vi "JL_Parse_Snapshot.vi"(0 "GEA2 Reference In":refnum<k24>, 5 "GEA Inputs":T2={"Source"=228, "Destination"=192} {"Destination" format="%.0x"; "Source" format="%.0x"}, 7 "SnapShot Location":T1={"ERD Number"=57629, "Data Type"=enum."string"} {"ERD Number" format="%.0x"}, 11 "Error In":errorcluster, 12 "Low Level Tries":u8=5) -> (4 "GEA2 Reference Out":refnum<k24>, 8 "Fault Snapshot":string[](array[string]), 15 "Error Out":errorcluster)   [LabVIEW 2023]
uses:
  D:/Common/LabVIEW GEA2 Toolkit/source/GEA3 DLL Source/GeaCommunication.dll
  Common/LabVIEW GEA2 Toolkit/source/GEA3 DLL Source/GeaCommunication.dll
  Common/LabVIEW GEA2 Toolkit/GEA3/type defs/Source_Destination.ctl
  Common/LabVIEW GEA2 Toolkit/GEA3/type defs/ERD Read Data In.ctl
  Common/LabVIEW GEA2 Toolkit/GEA3/library/GEA2_Toolkit.lvlib
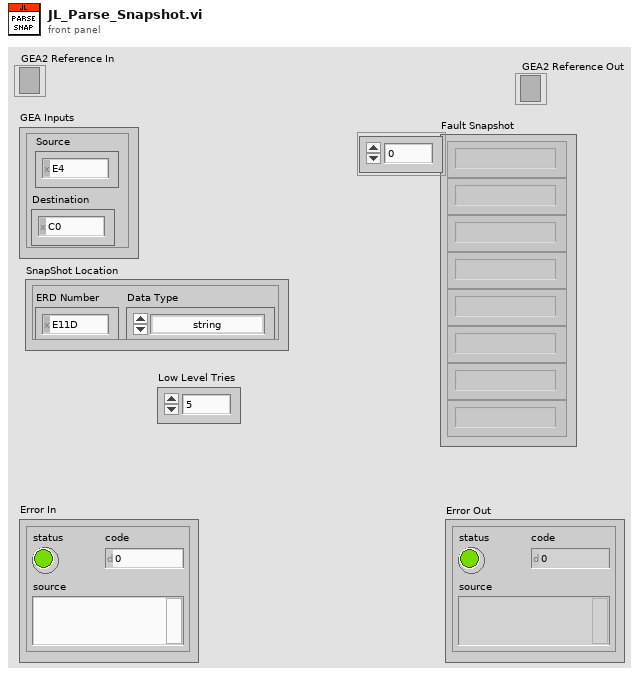
[diagram p1: front panel]
types:
  T1 = typedef "ERD Read Data In.ctl" = cluster{"ERD Number":u16, "Data Type":enum16{"string", "boolean", "uint8_t", "uint16_t", "uint32_t", "uint64_t", "int8_t", "int16_t", "int32_t", "int64_t"}}
  T2 = typedef "Source_Destination.ctl" = cluster{"Source":u8, "Destination":u8}
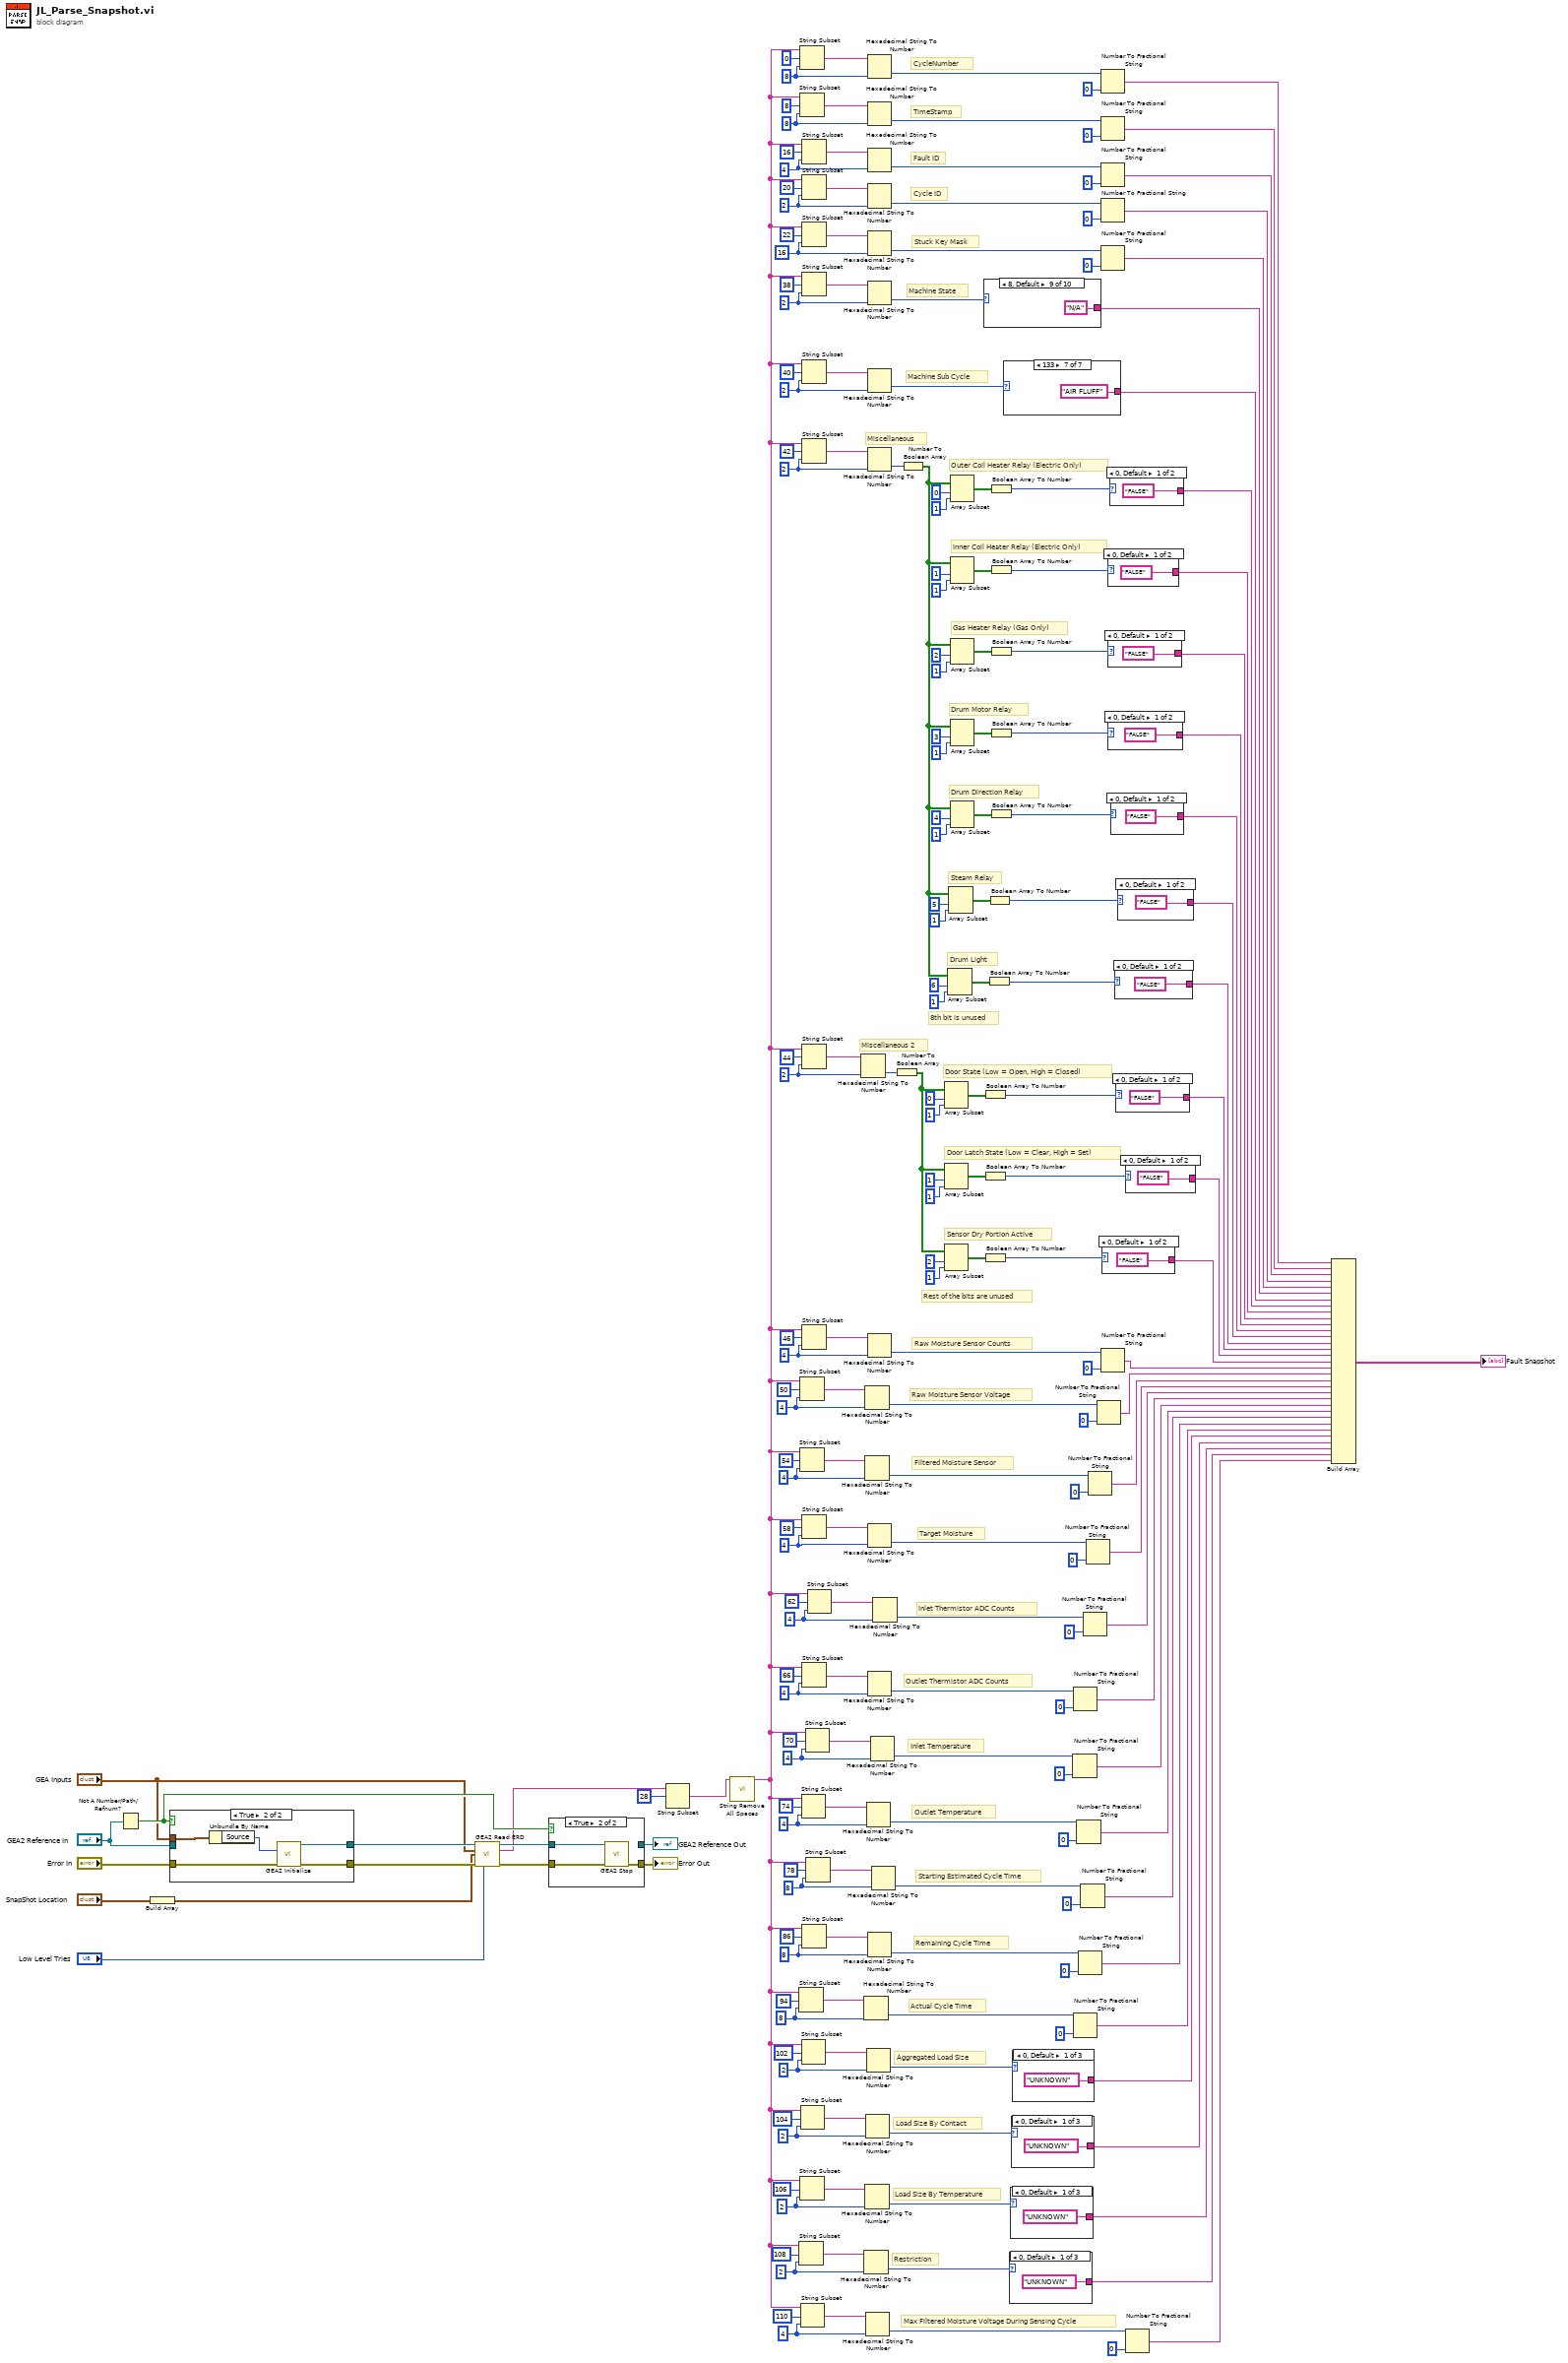
[diagram p0: block diagram]
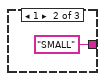
[diagram p2: hidden frame]
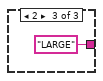
[diagram p3: hidden frame]
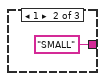
[diagram p4: hidden frame]
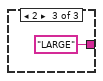
[diagram p5: hidden frame]
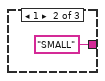
[diagram p6: hidden frame]
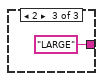
[diagram p7: hidden frame]
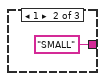
[diagram p8: hidden frame]
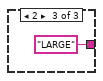
[diagram p9: hidden frame]
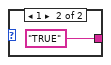
[diagram p10: hidden frame]
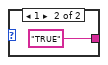
[diagram p11: hidden frame]
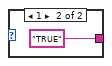
[diagram p12: hidden frame]
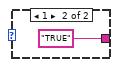
[diagram p13: hidden frame]
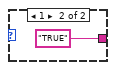
[diagram p14: hidden frame]
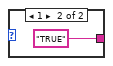
[diagram p15: hidden frame]
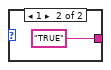
[diagram p16: hidden frame]
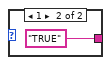
[diagram p17: hidden frame]
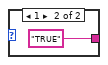
[diagram p18: hidden frame]
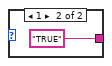
[diagram p19: hidden frame]
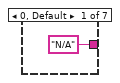
[diagram p20: hidden frame]
diagram:
  w14 = 4 ("length (rest)")
  w18 = 2 ("length (rest)")
  w22 = 2 ("length (rest)")
  w26 = 2 ("length (rest)")
  w31 = 2 ("length (rest)")
  w122 = 8 ("length (rest)")
  w123 = 4 ("length (rest)")
  w130 = 4 ("length (rest)")
  w146 = 8 ("length (rest)")
  w147 = 8 ("length (rest)")
  w148 = 4 ("length (rest)")
  w149 = 4 ("length (rest)")
  w150 = 4 ("length (rest)")
  w151 = 4 ("length (rest)")
  w152 = 4 ("length (rest)")
  w153 = 4 ("length (rest)")
  w63 = 2 ("length (rest)")
  w154 = 2 ("length (rest)")
  w155 = 2 ("length (rest)")
  w156 = 2 ("length (rest)")
  w157 = 16 ("length (rest)")
  w158 = 2 ("length (rest)")
  w159 = 4 ("length (rest)")
  w160 = 8 ("length (rest)")
  w161 = 8 ("length (rest)")
  # "Max Filtered Moisture Voltage During Sensing Cycle"
  # "Restriction"
  # "Load Size By Temperature"
  # "Load Size By Contact"
  # "Aggregated Load Size"
  # "Actual Cycle Time"
  # "Remaining Cycle Time"
  # "Starting Estimated Cycle Time"
  # "Outlet Temperature"
  # "Inlet Temperature"
  # "Outlet Thermistor ADC Counts"
  # "Inlet Thermistor ADC Counts"
  # "Target Moisture"
  # "Filtered Moisture Sensor"
  # "Rest of the bits are unused"
  # "Sensor Dry Portion Active"
  # "Door Latch State (Low = Clear, High = Set)"
  # "Door State (Low = Open, High = Closed)"
  # "Miscellaneous 2"
  # "8th bit is unused"
  # "Drum Light"
  # "Steam Relay"
  # "Drum Direction Relay"
  # "Drum Motor Relay"
  # "Gas Heater Relay (Gas Only)"
  # "Inner Coil Heater Relay (Electric Only)"
  # "Outer Coil Heater Relay (Electric Only)"
  # "Stuck Key Mask"
  # "Raw Moisture Sensor Counts"
  # "Raw Moisture Sensor Voltage"
  # "Miscellaneous"
  # "Machine Sub Cycle"
  # "Cycle ID"
  # "Fault ID"
  # "Machine State"
  # "TimeStamp"
  # "CycleNumber"
  n1 = Not A Number/Path/Refnum?(number/path/refnum="GEA2 Reference In") -> (NaN/Path/Refnum?=w142:bool)
  n2 = Build Array("SnapShot Location") -> (w1:T1[])
  n3 = case shown="True" w142 {
    tunnel: "GEA Inputs" -> [_ w217]
    tunnel: "Error In" -> [w212 w216]
    tunnel: [w212 w215] -> w136
    tunnel: [w211 w214] -> w140
    tunnel: "GEA2 Reference In" -> [w211 _]
    frame False {
    }
    frame True {
      n4 = Unbundle By Name(w217) -> ("Source"=w213:u8)
      n5 = call "GEA2 Initialize.vi"("Source Address"=w213, "error in"=w216) -> ("GEA2 Reference Out"=w214:refnum<k24>, "error out"=w215:errorcluster)  [unwired: 10 in, 2 out]
    }
  }
  n6 = call "GEA2 Read ERD.vi"("GEA2 Reference In"=w140, "GEA Inputs"="GEA Inputs", "Read ERD List"=w1, "Error In"=w136, "Low Level Tries"="Low Level Tries") -> ("GEA2 Reference Out"=w138:refnum<k24>, "Raw Data Out"=w131:string, "Error Out"=w137:errorcluster)  [unwired: 7 in, 1 out]
  n7 = case shown="True" w142 {
    tunnel: [w218 w222] -> w143
    tunnel: [w219 _] -> w141
    tunnel: w138 -> [w219 w220]
    tunnel: w137 -> [w218 w221]
    frame False {
    }
    frame True {
      n8 = call "GEA2 Stop.vi"("GEA2 Reference In"=w220, "Error In"=w221) -> ("Error Out"=w222:errorcluster)  [unwired: 13 in]
    }
  }
  "Error Out" <- w143
  "GEA2 Reference Out" <- w141
  n9 = String Subset(string=w131, offset (0)=28) -> (substring=w132:string)  [unwired: 1 in]
  n10 = call "String Remove All Spaces.vi"("Input String"=w132) -> ("Spaces Removed"=w9:string)  [unwired: 13 in, 1 out]
  n11 = String Subset(string=w9, offset (0)=94, length (rest)=w122) -> (substring=w121:string)
  n12 = String Subset(string=w9, offset (0)=108, length (rest)=w18) -> (substring=w17:string)
  n13 = String Subset(string=w9, offset (0)=0, length (rest)=w161) -> (substring=w210:string)
  n14 = String Subset(string=w9, offset (0)=8, length (rest)=w160) -> (substring=w209:string)
  n15 = String Subset(string=w9, offset (0)=50, length (rest)=w130) -> (substring=w129:string)
  n16 = String Subset(string=w9, offset (0)=54, length (rest)=w123) -> (substring=w124:string)
  n17 = String Subset(string=w9, offset (0)=106, length (rest)=w22) -> (substring=w21:string)
  n18 = String Subset(string=w9, offset (0)=104, length (rest)=w26) -> (substring=w25:string)
  n19 = String Subset(string=w9, offset (0)=110, length (rest)=w14) -> (substring=w13:string)
  n20 = String Subset(string=w9, offset (0)=74, length (rest)=w148) -> (substring=w184:string)
  n21 = String Subset(string=w9, offset (0)=102, length (rest)=w31) -> (substring=w30:string)
  n22 = String Subset(string=w9, offset (0)=16, length (rest)=w159) -> (substring=w208:string)
  n23 = String Subset(string=w9, offset (0)=20, length (rest)=w158) -> (substring=w207:string)
  n24 = String Subset(string=w9, offset (0)=22, length (rest)=w157) -> (substring=w196:string)
  n25 = String Subset(string=w9, offset (0)=38, length (rest)=w156) -> (substring=w197:string)
  n26 = String Subset(string=w9, offset (0)=40, length (rest)=w155) -> (substring=w198:string)
  n27 = String Subset(string=w9, offset (0)=42, length (rest)=w154) -> (substring=w3:string)
  n28 = String Subset(string=w9, offset (0)=44, length (rest)=w63) -> (substring=w64:string)
  n29 = String Subset(string=w9, offset (0)=46, length (rest)=w153) -> (substring=w185:string)
  n30 = String Subset(string=w9, offset (0)=58, length (rest)=w152) -> (substring=w195:string)
  n31 = String Subset(string=w9, offset (0)=66, length (rest)=w150) -> (substring=w193:string)
  n32 = String Subset(string=w9, offset (0)=86, length (rest)=w146) -> (substring=w182:string)
  n33 = String Subset(string=w9, offset (0)=70, length (rest)=w149) -> (substring=w192:string)
  n34 = String Subset(string=w9, offset (0)=78, length (rest)=w147) -> (substring=w183:string)
  n35 = String Subset(string=w9, offset (0)=62, length (rest)=w151) -> (substring=w194:string)
  n36 = Hexadecimal String To Number(string=w64, default (0uL)=w63) -> (number=w78:i32)  [unwired: 1 in, 1 out]
  n37 = Hexadecimal String To Number(string=w121, default (0uL)=w122) -> (number=w32:i32)  [unwired: 1 in, 1 out]
  n38 = Hexadecimal String To Number(string=w17, default (0uL)=w18) -> (number=w15:i32)  [unwired: 1 in, 1 out]
  n39 = Hexadecimal String To Number(string=w129, default (0uL)=w130) -> (number=w126:i32)  [unwired: 1 in, 1 out]
  n40 = Hexadecimal String To Number(string=w124, default (0uL)=w123) -> (number=w56:i32)  [unwired: 1 in, 1 out]
  n41 = Hexadecimal String To Number(string=w21, default (0uL)=w22) -> (number=w19:i32)  [unwired: 1 in, 1 out]
  n42 = Hexadecimal String To Number(string=w25, default (0uL)=w26) -> (number=w23:i32)  [unwired: 1 in, 1 out]
  n43 = Hexadecimal String To Number(string=w13, default (0uL)=w14) -> (number=w10:i32)  [unwired: 1 in, 1 out]
  n44 = Hexadecimal String To Number(string=w184, default (0uL)=w148) -> (number=w41:i32)  [unwired: 1 in, 1 out]
  n45 = Hexadecimal String To Number(string=w30, default (0uL)=w31) -> (number=w27:i32)  [unwired: 1 in, 1 out]
  n46 = Hexadecimal String To Number(string=w210, default (0uL)=w161) -> (number=w173:i32)  [unwired: 1 in, 1 out]
  n47 = Hexadecimal String To Number(string=w209, default (0uL)=w160) -> (number=w174:i32)  [unwired: 1 in, 1 out]
  n48 = Hexadecimal String To Number(string=w208, default (0uL)=w159) -> (number=w162:i32)  [unwired: 1 in, 1 out]
  n49 = Hexadecimal String To Number(string=w207, default (0uL)=w158) -> (number=w171:i32)  [unwired: 1 in, 1 out]
  n50 = Hexadecimal String To Number(string=w196, default (0uL)=w157) -> (number=w172:i32)  [unwired: 1 in, 1 out]
  n51 = Hexadecimal String To Number(string=w197, default (0uL)=w156) -> (number=w119:i32)  [unwired: 1 in, 1 out]
  n52 = Hexadecimal String To Number(string=w198, default (0uL)=w155) -> (number=w117:i32)  [unwired: 1 in, 1 out]
  n53 = Hexadecimal String To Number(string=w3, default (0uL)=w154) -> (number=w115:i32)  [unwired: 1 in, 1 out]
  n54 = Hexadecimal String To Number(string=w185, default (0uL)=w153) -> (number=w170:i32)  [unwired: 1 in, 1 out]
  n55 = Hexadecimal String To Number(string=w195, default (0uL)=w152) -> (number=w53:i32)  [unwired: 1 in, 1 out]
  n56 = Hexadecimal String To Number(string=w193, default (0uL)=w150) -> (number=w47:i32)  [unwired: 1 in, 1 out]
  n57 = Hexadecimal String To Number(string=w182, default (0uL)=w146) -> (number=w35:i32)  [unwired: 1 in, 1 out]
  n58 = Hexadecimal String To Number(string=w192, default (0uL)=w149) -> (number=w44:i32)  [unwired: 1 in, 1 out]
  n59 = Hexadecimal String To Number(string=w183, default (0uL)=w147) -> (number=w38:i32)  [unwired: 1 in, 1 out]
  n60 = Hexadecimal String To Number(string=w194, default (0uL)=w151) -> (number=w50:i32)  [unwired: 1 in, 1 out]
  n61 = Number To Boolean Array(number=w78) -> (Boolean array=w65:bool[])
  n62 = Number To Boolean Array(number=w115) -> (Boolean array=w86:bool[])
  n63 = Array Subset(array=w65, index=0, length=1) -> (w68:bool[])
  n64 = Array Subset(array=w65, index=1, length=1) -> (w67:bool[])
  n65 = Array Subset(array=w65, index=2, length=1) -> (w66:bool[])
  n66 = Array Subset(array=w86, index=6, length=1) -> (w87:bool[])
  n67 = Array Subset(array=w86, index=5, length=1) -> (w91:bool[])
  n68 = Array Subset(array=w86, index=0, length=1) -> (w99:bool[])
  n69 = Array Subset(array=w86, index=1, length=1) -> (w98:bool[])
  n70 = Array Subset(array=w86, index=2, length=1) -> (w97:bool[])
  n71 = Array Subset(array=w86, index=3, length=1) -> (w96:bool[])
  n72 = Array Subset(array=w86, index=4, length=1) -> (w95:bool[])
  n73 = case shown="8, Default" w119 {
    tunnel: ["IDLE" "STANDBY" "RUN" "PAUSE" "EOC" "DSM DELAY RUN" "DELAY RUN" "DELAY PAUSE" "N/A" "CLEAN SPEAK"] -> w118
    frame 0 {
    }
    frame 1 {
    }
    frame 2 {
    }
    frame 3 {
    }
    frame 4 {
    }
    frame 5 {
    }
    frame 6 {
    }
    frame 7 {
    }
    frame 8, Default {
    }
    frame 128 {
    }
  }
  n74 = Boolean Array To Number(Boolean array=w68) -> (number=w77:u32)
  n75 = Boolean Array To Number(Boolean array=w67) -> (number=w76:u32)
  n76 = Boolean Array To Number(Boolean array=w66) -> (number=w75:u32)
  n77 = Boolean Array To Number(Boolean array=w87) -> (number=w90:u32)
  n78 = Boolean Array To Number(Boolean array=w91) -> (number=w94:u32)
  n79 = Boolean Array To Number(Boolean array=w99) -> (number=w114:u32)
  n80 = Boolean Array To Number(Boolean array=w98) -> (number=w113:u32)
  n81 = Boolean Array To Number(Boolean array=w97) -> (number=w112:u32)
  n82 = Boolean Array To Number(Boolean array=w96) -> (number=w111:u32)
  n83 = Boolean Array To Number(Boolean array=w95) -> (number=w110:u32)
  n84 = case shown="133" w117 {
    tunnel: ["N/A" "DRYING" "MIST STEAM" "COOL DOWN" "EXTENDED TUMBLE" "DAMP" "AIR FLUFF"] -> w116
    frame 0, Default {
    }
    frame 128 {
    }
    frame 129 {
    }
    frame 130 {
    }
    frame 131 {
    }
    frame 132 {
    }
    frame 133 {
    }
  }
  n85 = case shown="0, Default" w15 {
    tunnel: ["UNKNOWN" "SMALL" "LARGE"] -> w5
    frame 0, Default {
    }
    frame 1 {
    }
    frame 2 {
    }
  }
  n86 = case shown="0, Default" w19 {
    tunnel: ["UNKNOWN" "SMALL" "LARGE"] -> w6
    frame 0, Default {
    }
    frame 1 {
    }
    frame 2 {
    }
  }
  n87 = case shown="0, Default" w23 {
    tunnel: ["UNKNOWN" "SMALL" "LARGE"] -> w7
    frame 0, Default {
    }
    frame 1 {
    }
    frame 2 {
    }
  }
  n88 = case shown="0, Default" w27 {
    tunnel: ["UNKNOWN" "SMALL" "LARGE"] -> w8
    frame 0, Default {
    }
    frame 1 {
    }
    frame 2 {
    }
  }
  n89 = Number To Fractional String(number=w44, precision (6)=i16 0) -> (F-format string=w43:string)  [unwired: 2 in]
  n90 = Number To Fractional String(number=w47, precision (6)=i16 0) -> (F-format string=w46:string)  [unwired: 2 in]
  n91 = Number To Fractional String(number=w32, precision (6)=i16 0) -> (F-format string=w28:string)  [unwired: 2 in]
  n92 = Number To Fractional String(number=w41, precision (6)=i16 0) -> (F-format string=w40:string)  [unwired: 2 in]
  n93 = Number To Fractional String(number=w35, precision (6)=i16 0) -> (F-format string=w34:string)  [unwired: 2 in]
  n94 = Number To Fractional String(number=w38, precision (6)=i16 0) -> (F-format string=w37:string)  [unwired: 2 in]
  n95 = Number To Fractional String(number=w50, precision (6)=i16 0) -> (F-format string=w49:string)  [unwired: 2 in]
  n96 = Number To Fractional String(number=w53, precision (6)=i16 0) -> (F-format string=w52:string)  [unwired: 2 in]
  n97 = Number To Fractional String(number=w56, precision (6)=i16 0) -> (F-format string=w55:string)  [unwired: 2 in]
  n98 = Number To Fractional String(number=w126, precision (6)=i16 0) -> (F-format string=w58:string)  [unwired: 2 in]
  n99 = Number To Fractional String(number=w173, precision (6)=u32 0) -> (F-format string=w169:string)  [unwired: 2 in]
  n100 = Number To Fractional String(number=w174, precision (6)=u32 0) -> (F-format string=w168:string)  [unwired: 2 in]
  n101 = Number To Fractional String(number=w162, precision (6)=u32 0) -> (F-format string=w163:string)  [unwired: 2 in]
  n102 = Number To Fractional String(number=w171, precision (6)=u32 0) -> (F-format string=w167:string)  [unwired: 2 in]
  n103 = Number To Fractional String(number=w172, precision (6)=i16 0) -> (F-format string=w166:string)  [unwired: 2 in]
  n104 = Number To Fractional String(number=w170, precision (6)=i16 0) -> (F-format string=w59:string)  [unwired: 2 in]
  n105 = case shown="0, Default" w75 {
    tunnel: ["FALSE" "TRUE"] -> w60
    frame 0, Default {
    }
    frame 1 {
    }
  }
  n106 = case shown="0, Default" w113 {
    tunnel: ["FALSE" "TRUE"] -> w84
    frame 0, Default {
    }
    frame 1 {
    }
  }
  n107 = case shown="0, Default" w112 {
    tunnel: ["FALSE" "TRUE"] -> w83
    frame 0, Default {
    }
    frame 1 {
    }
  }
  n108 = case shown="0, Default" w111 {
    tunnel: ["FALSE" "TRUE"] -> w82
    frame 0, Default {
    }
    frame 1 {
    }
  }
  n109 = case shown="0, Default" w114 {
    tunnel: ["FALSE" "TRUE"] -> w85
    frame 0, Default {
    }
    frame 1 {
    }
  }
  n110 = case shown="0, Default" w110 {
    tunnel: ["FALSE" "TRUE"] -> w81
    frame 0, Default {
    }
    frame 1 {
    }
  }
  n111 = case shown="0, Default" w90 {
    tunnel: ["FALSE" "TRUE"] -> w79
    frame 0, Default {
    }
    frame 1 {
    }
  }
  n112 = case shown="0, Default" w77 {
    tunnel: ["FALSE" "TRUE"] -> w62
    frame 0, Default {
    }
    frame 1 {
    }
  }
  n113 = case shown="0, Default" w94 {
    tunnel: ["FALSE" "TRUE"] -> w80
    frame 0, Default {
    }
    frame 1 {
    }
  }
  n114 = case shown="0, Default" w76 {
    tunnel: ["FALSE" "TRUE"] -> w61
    frame 0, Default {
    }
    frame 1 {
    }
  }
  n115 = Number To Fractional String(number=w10, precision (6)=i16 0) -> (F-format string=w4:string)  [unwired: 2 in]
  n116 = Build Array(w169, w168, w163, w167, w166, w118, w116, w85, w84, w83, w82, w81, w80, w79, w62, w61, w60, w59, w58, w55, w52, w49, w46, w43, w40, w37, w34, w28, w8, w7, w6, w5, w4) -> (→"Fault Snapshot":string[])
